vi "LVFunction_Imop_Compute_PSF from HasoField.vi"(0 "HasoField in":refnum<class "HasoField.lvclass">, 5 "Surface PSF":refnum<class "SurfaceFloat.lvclass">, 7 "Path":path, 9 "param":T1={"null_phase"=TRUE, "flat_intensity"=TRUE}, 11 "error in (no error)":errorcluster, 12 "defocus":sgl) -> (4 "HasoField out":refnum<class "HasoField.lvclass">, 6 "Surface PSF":refnum<class "SurfaceFloat.lvclass">, 15 "error out":errorcluster)   [LabVIEW 2020]
doc: "Point spread function.\n\n--------------------------------------------------------------------------------\n\n<B>HasoFieldIn</B> : HasoField object.\n\n<B>HasoFieldOut</B> : HasoField object.\n\n<B>null_phase</B> : Phase is null.\n\n<B>flat_intensity</B> : Intensity surface is flat.\n\n<B>defocus</B> : Defocus parameter.\n\n<B>config_file_path</B> : Absolute path to the Haso configuration file.\n\n<B>SurfacePSF</B> : PSF stored as cSurface.\n\n<B>ErrorIn</B> : Error\n\n<B>ErrorOut</B> : Error"
uses:
  HasoField.lvclass
  SurfaceFloat.lvclass
  LVClasse_SurfaceFloat Read SurfaceFloat.vi
  LVClass_HasoField Read HasoField.vi
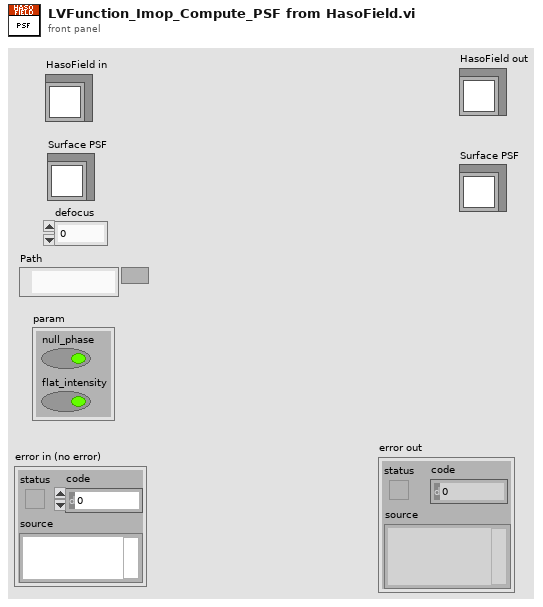
[diagram p1: front panel]
types:
  T1 = cluster{"null_phase":bool, "flat_intensity":bool}
  T2 = typedef "ClassID.ctl" = i64
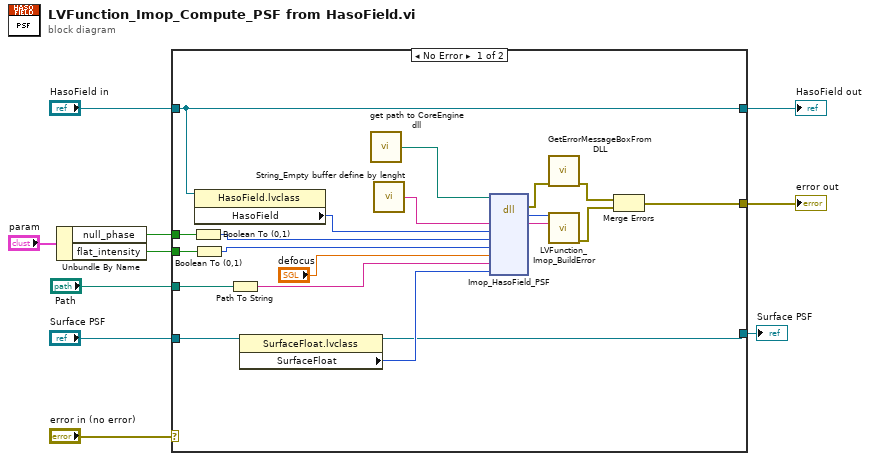
[diagram p0: block diagram]
diagram:
  n1 = Unbundle By Name("param") -> ("null_phase"=w4:bool, "flat_intensity"=w3:bool)
  n2 = case shown="No Error" "error in (no error)" {
    selector: "error in (no error)" -> [_ w33]
    tunnel: [w23 w33] -> w9
    tunnel: [w20 w32] -> w7
    tunnel: "HasoField in" -> [w20 w32]
    tunnel: "Path" -> [w22 _]
    tunnel: w4 -> [w18 _]
    tunnel: w3 -> [w17 _]
    tunnel: "Surface PSF" -> [w13 w31]
    tunnel: [w11 w31] -> w1
    frame No Error {
      n3 = Boolean To (0,1)(Boolean=w18) -> (0, 1=w16:i16)
      n4 = Boolean To (0,1)(Boolean=w17) -> (0, 1=w15:i16)
      n5 = property class="HasoField.lvclass"(reference=w20) -> ("HasoField"=w19:T2)  [unwired: 1 in, 2 out]
      n6 = Path To String(path=w22) -> (string=w21:string)
      n7 = property class="SurfaceFloat.lvclass"(reference=w13) -> (reference out=w11:refnum<class "SurfaceFloat.lvclass">, "SurfaceFloat"=w12:T2)  [unwired: 1 in, 1 out]
      n8 = call "get path to CoreEngine dll.vi"() -> ("path to wavekit library"=w27:path)  [unwired: 14 in, 1 out]
      n9 = call "String_Empty buffer define by lenght.vi"() -> ("Empty buffer"=w30:string)  [unwired: 1 in]
      n10 = dll-call lib="D:/2_trunk/Soft_haso/ImOpCoreEngine4_LV2011/DLLs/ImopEngine4_vc100.dll" fn="Imop_HasoField_PSF"(path in=w27, "message"=w30, "hasofield"=w19, "null_phase"=w16, "flat_intensity"=w15, "defocus"="defocus", "config_file_path"=w21, "SWP_psf"=w12) -> (error out=w26:errorcluster, "return type"=w28:i32, "message"=w29:string)  [unwired: 8 in, 1 out]
      n11 = call "GetErrorMessageBoxFromDLL.vi"("error IN"=w26) -> ("error OUT"=w25:errorcluster)  [unwired: 10 in]
      n12 = call "LVFunction_Imop_BuildError.vi"("code"=w28, "String to Prepend to source (\"\")"=w29) -> ("error out"=w24:errorcluster)  [unwired: 13 in]
      n13 = Merge Errors(w25, w24) -> (w23:errorcluster)
    }
    frame Error {
    }
  }
  "error out" <- w9
  "HasoField out" <- w7
  "Surface PSF" <- w1
